vi "Pre Launch Init.vi"(11 "ATM Controller in":refnum<class "Sim User Console Actor.lvclass">) -> (0 "error out":errorcluster, 3 "ATM Controller out":refnum<class "Sim User Console Actor.lvclass">)   [LabVIEW 2019, in "Sim User Console Actor.lvlib" / "Sim User Console Actor.lvclass"]
doc: "(<B>Filename</B>: Actor Framework.lvlib:Actor.lvclass:Pre Launch Init.vi)\n\nDefines behavior that occurs after the Launch Nested Actor method is invoked but before the actor's Actor Core method begins running.\n\nBy default, this method does nothing. A descendant class may override it to define behavior."
uses:
  Sim User Console Actor.lvclass
  Sim User Console Actor.lvclass/Sim User Console Actor.ctl
  User Console Actor/User Console Actor/User Console Actor.lvclass
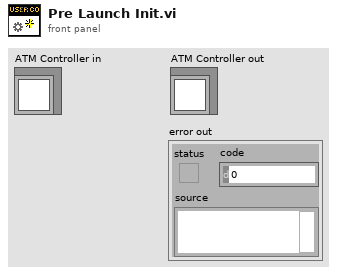
[diagram p1: front panel]
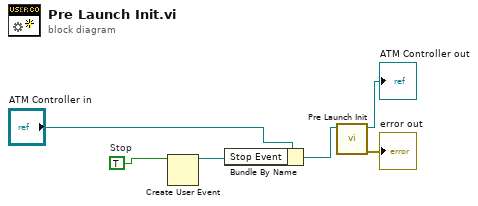
[diagram p0: block diagram]
diagram:
  w4 = TRUE  # Stop
  n1 = Create User Event(user event datatype=w4) -> (user event=w1:refnum<user-event>)  [unwired: 1 in, 1 out]
  n2 = Bundle By Name(cluster="ATM Controller in", "Stop Event"=w1) -> (w2:refnum<class "Sim User Console Actor.lvclass">)
  n3 = call-parent "Pre Launch Init.vi"("Actor in"=w2) -> ("error out"=→"error out":errorcluster, "Actor out"=→"ATM Controller out":refnum<class "Sim User Console Actor.lvclass">)  [unwired: 9 in]
